vi "Launch as Nested.vi"(8 "error in (no error)":errorcluster, 9 "Group Config":refnum<class "Group.lvclass">, 10 "DataProcessor Config":refnum<class "Config Element.lvclass">, 11 "Parent Task in":refnum<class "Task.lvclass">) -> (0 "error out":errorcluster, 2 "API":refnum<class "DataHandlerAPI.lvclass">, 3 "Parent Task":refnum<class "Task.lvclass">)   [LabVIEW 2020, in "VolatusData.lvlib" / "DataProcessor.lvclass"]
uses:
  DataProcessor.lvclass
  DataProcessor.lvclass/DataProcessor.ctl
  Volatus/Task/Task.lvclass
  DataHandlerAPI/DataHandlerAPI.lvclass
  C:/dev/lv20CE/relink/lv-volatus/VolatusData/DataHandlerTask/DataHandlerTask.lvclass
  C:/dev/lv20CE/relink/lv-volatus/Volatus/Task/Task.lvclass
  C:/Program Files (x86)/National Instruments/LabVIEW 2020/vi.lib/ActorFramework/Actor/Actor.lvclass
  C:/dev/lv20CE/relink/lv-volatus/Volatus/TaskStateHandler/TaskStateHandler.lvclass
  C:/dev/lv20CE/relink/lv-volatus/Volatus/VectoMessageHandler/VectoMessageHandler.lvclass
  C:/dev/lv20CE/relink/lv-volatus/Volatus/API Provider/API Provider.lvclass
  C:/dev/lv20CE/relink/lv-volatus/VolatusData/DataHandler/DataHandler.lvclass
  C:/dev/lv20CE/relink/lv-volatus/VolatusData/DataProcessor/DataProcessor.lvclass
  C:/dev/lv20CE/relink/lv-volatus/Volatus/Abortable/Abortable.lvclass
  C:/dev/lv20CE/relink/lv-volatus/Volatus/Reconfigurable/Reconfigurable.lvclass
  DataHandlerTask/DataHandlerTask.lvclass
  C:/dev/lv20CE/relink/lv-volatus/VolatusData/DataHandlerAPI/DataHandlerAPI.lvclass
  C:/dev/lv20CE/relink/lv-volatus/Volatus/API/API.lvclass
  VolatusConfig/Group/Group.lvclass
  lv-cdm/CDM-Config/Config Element/Config Element.lvclass
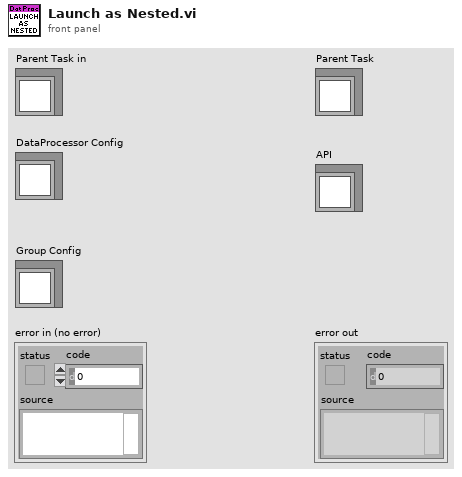
[diagram p1: front panel]
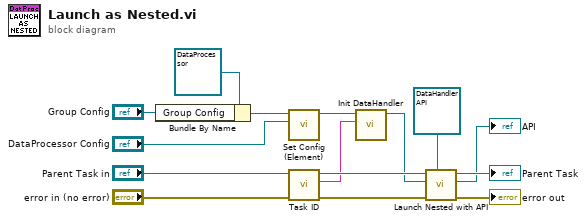
[diagram p0: block diagram]
diagram:
  n1 = Bundle By Name(cluster=refnum<class "DataProcessor.lvclass"> refnum ("Volatus:DataProcessor.lvclass"), "Group Config"="Group Config") -> (w1:refnum<class "DataProcessor.lvclass">)
  n2 = call "Set Config (Element).vi"("Config Element"="DataProcessor Config", "Task in"=w1) -> ("Task out"=w3:refnum<class "DataProcessor.lvclass">)  [unwired: 8 in, 1 out]
  n3 = call-dynamic "Task ID.vi"("error in (no error)"="error in (no error)", "Task in"="Parent Task in") -> ("error out"=w9:errorcluster, "Task ID"=w6:string, "Task out"=w11:refnum<class "Task.lvclass">)  [unwired: 7 in]
  n4 = call "Init DataHandler.vi"("Parent Name"=w6, "DataHandlerTask in"=w3) -> ("DataHandlerTask out"=w7:refnum<class "DataProcessor.lvclass">)  [unwired: 8 in, 1 out]
  n5 = call "Launch Nested with API.vi"("API Type"=refnum<class "DataHandlerAPI.lvclass"> refnum ("Volatus:DataHandlerAPI"), "error in (no error)"=w9, "Nested Task"=w7, "Task in"=w11) -> ("error out"=→"error out":errorcluster, "API"=→"API":refnum<class "DataHandlerAPI.lvclass">, "Task out"=→"Parent Task":refnum<class "Task.lvclass">)  [unwired: 5 in]
